vi "Configure Multitone Frequency.vi"(6 "Phase Distribution Algorithm (0: mpZero)":i32(ring) items=["mpZero", "mpNewman", "mpSchroeder", "mpZygmund", "mpRudin", "mpRandom"], 7 "Tone Distribution Algorithm (0: mfLinear)":i32(ring) items=["mfLinear", "mfLog", "mfOctave", "mfDecade", "mfPrime", "mfLinearPrime", "mfLogPrime"], 8 "error in (no error)":errorcluster, 9 "Stop Frequency (30 Hz)":dbl=30.0, 10 "Start Frequency (30 Hz)":dbl=30.0, 11 "VISA resource name":refnum<visa-resource-name>) -> (0 "error out":errorcluster, 3 "VISA resource name out":refnum<visa-resource-name>)   [LabVIEW 2014, in "Stanford Research SR1.lvlib"]
doc: "Configures the attributes for the Multitone Frequency."
uses:
  Stanford Research SR1.lvlib
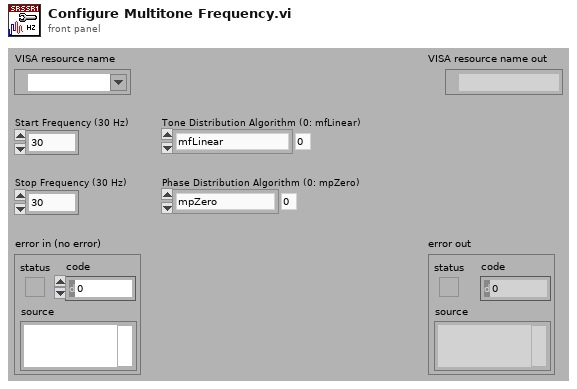
[diagram p1: front panel]
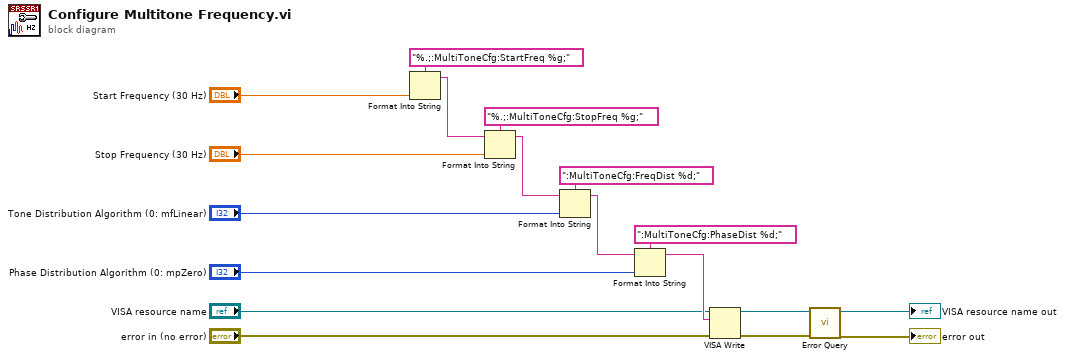
[diagram p0: block diagram]
diagram:
  n1 = Format Into String(format string="%.;:MultiToneCfg:StartFreq %g;", "Start Frequency (30 Hz)") -> (resulting string=w16:string)  [unwired: 2 in, 1 out]
  n2 = Format Into String(format string="%.;:MultiToneCfg:StopFreq %g;", initial string=w16, "Stop Frequency (30 Hz)") -> (resulting string=w13:string)  [unwired: 1 in, 1 out]
  n3 = Format Into String(format string=":MultiToneCfg:FreqDist %d;", initial string=w13, "Tone Distribution Algorithm (0: mfLinear)") -> (resulting string=w10:string)  [unwired: 1 in, 1 out]
  n4 = Format Into String(format string=":MultiToneCfg:PhaseDist %d;", initial string=w10, "Phase Distribution Algorithm (0: mpZero)") -> (resulting string=w7:string)  [unwired: 1 in, 1 out]
  n5 = VISA Write(VISA resource name="VISA resource name", write buffer=w7, error in (no error)="error in (no error)") -> (VISA resource name out=w4:refnum<visa-resource-name>, error out=w3:errorcluster)  [unwired: 1 out]
  n6 = call "Error Query.vi"("error in (no error)"=w3, "VISA resource name"=w4) -> ("error out"=→"error out":errorcluster, "VISA resource name out"=→"VISA resource name out":refnum<visa-resource-name>)  [unwired: 6 in, 2 out]
